vi "Write Image Prefix.vi"(8 "error in (no error)":errorcluster, 10 "Prefix":string, 11 "HIJ Vision Application in":refnum<class "HIJ Vision Application.lvclass">) -> (0 "error out":errorcluster, 3 "HIJ Vision Application out":refnum<class "HIJ Vision Application.lvclass">)   [LabVIEW 2014, in "HIJ Vision Application.lvlib" / "HIJ Vision Application.lvclass"]
uses:
  HIJ Vision Application.lvclass
  HIJ Vision Application.lvclass/HIJ Vision Application.ctl
  Display Actors/HIJ Vision Display/HIJ Vision Display Messages/Write Image Name Prefix Msg/Write Image Name Prefix Msg.lvclass/Write Image Name Prefix Msg.ctl
  <vilib>/ActorFramework/Message Enqueuer/Message Enqueuer.lvclass/Message Enqueuer.ctl
  Read Display Enq.vi
  <vilib>/ActorFramework/Message Enqueuer/Enqueue.vi
  <vilib>/ActorFramework/Message Priority Queue/Priority Enqueue.vi
  <vilib>/ActorFramework/Message Enqueuer/Message Enqueuer.lvclass
  Display Actors/HIJ Vision Display/HIJ Vision Display Messages/Write Image Name Prefix Msg/Write Image Name Prefix Msg.lvclass
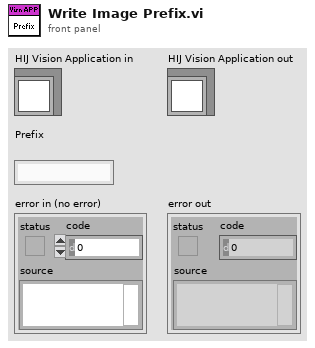
[diagram p1: front panel]
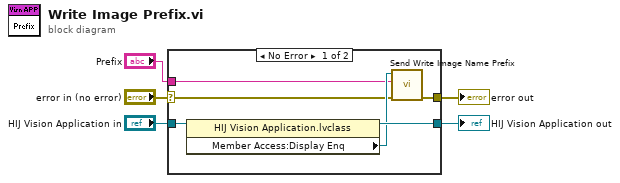
[diagram p0: block diagram]
diagram:
  n1 = case shown="No Error" "error in (no error)" {
    selector: "error in (no error)" -> [w7 w13]
    tunnel: [w6 w13] -> w4
    tunnel: [w10 w12] -> w2
    tunnel: "HIJ Vision Application in" -> [w11 w12]
    tunnel: "Prefix" -> [w8 _]
    frame No Error {
      n2 = property class="HIJ Vision Application.lvclass"(reference=w11) -> (reference out=w10:refnum<class "HIJ Vision Application.lvclass">, "Member Access:Display Enq"=w9:refnum<class "Message Enqueuer.lvclass">)  [unwired: 1 in, 1 out]
      n3 = call "Send Write Image Name Prefix.vi"("error in (no error)"=w7, "Image Name Prefix"=w8, "Message Enqueuer"=w9) -> ("error out"=w6:errorcluster)  [unwired: 7 in, 1 out]
    }
    frame Error {
    }
  }
  "error out" <- w4
  "HIJ Vision Application out" <- w2
